vi "IMS Stepper Move Scaled.vi"() -> ()   [LabVIEW 2021]
panel:
  in  "Scale Factor":dbl=-47.2441
  out "Position":dbl format="%.4f"
  out "error out":errorcluster
  in  "Mode":bool
  in  "Distance":dbl=1.0 min=-193273528.32 max=193273528.0 format="%.2f"
  in  "Instrument Address":refnum<visa-resource-name>
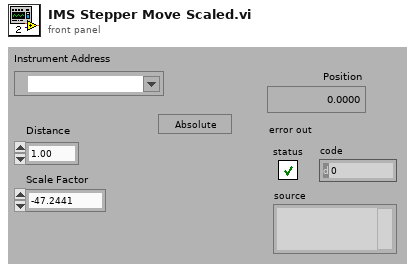
[diagram p1: front panel]
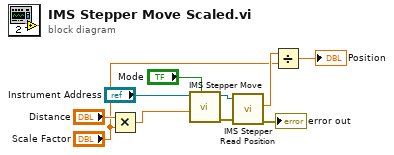
[diagram p0: block diagram]
diagram:
  n1 = Multiply(x="Distance", y="Scale Factor") -> (x*y=w5:dbl)
  n2 = call "IMS Stepper Move.vi"("Mode"="Mode", "Distance"=w5, "Instrument Address"="Instrument Address") -> ("error out"=w8:errorcluster, "Instrument Address Out"=w1:refnum<visa-resource-name>)  [unwired: 4 in]
  n3 = call "IMS Stepper Read Position.vi"("Instrument Address"=w1, "error in (no error)"=w8) -> ("Response"=w6:dbl, "error out"=→"error out":errorcluster)  [unwired: 2 in, 1 out]
  n4 = Divide(x=w6, y="Scale Factor") -> (x/y=→"Position":dbl)
